vi "ESC controller continuous.vi"() -> ()   [LabVIEW 2020]
panel:
  in  "Max. output (%)":sgl=100.0
  in  "Cool-down time (s)":sgl=60.0
  in  "end":bool
  out "Cool time":sgl(slide) caption="Cooling down...." scale=0.0..1.0
  in  "S-stop":bool
  in  "Output %":sgl(slide) min=0 max=20 scale=0.0..100.0
  in  "E-stop":bool
  out "Error out":errorcluster
  in  "Port":refnum<visa-resource-name>
  # "PN 15/02/2017"
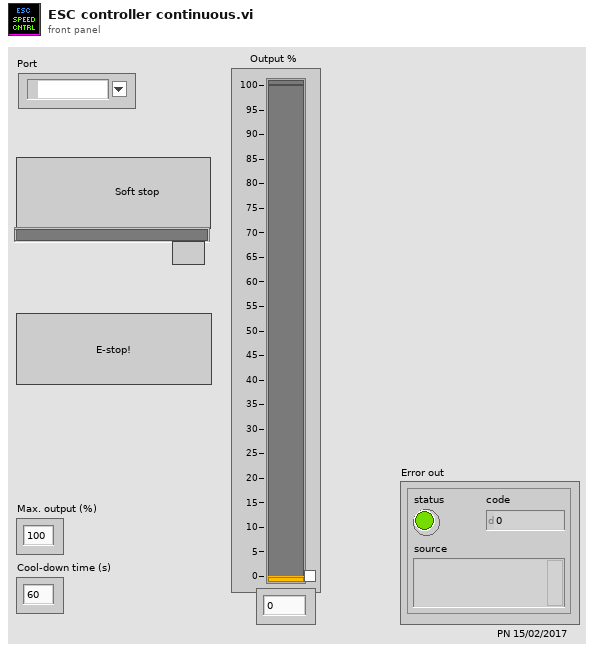
[diagram p1: front panel]
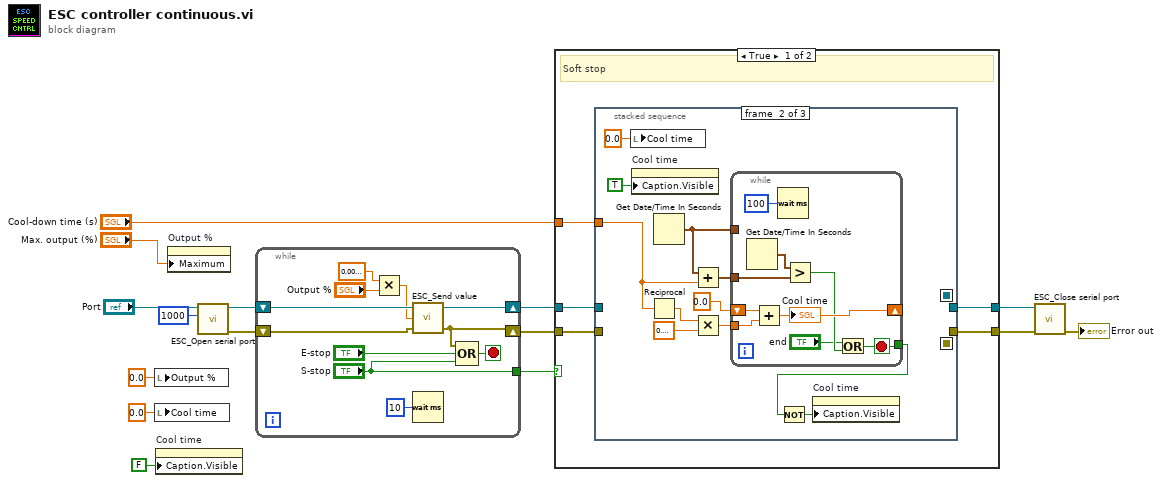
[diagram p0: block diagram]
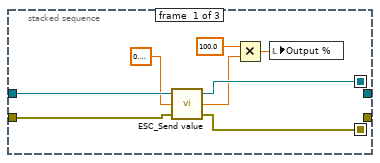
[diagram p2: hidden frame]
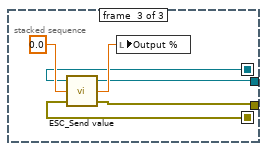
[diagram p3: hidden frame]
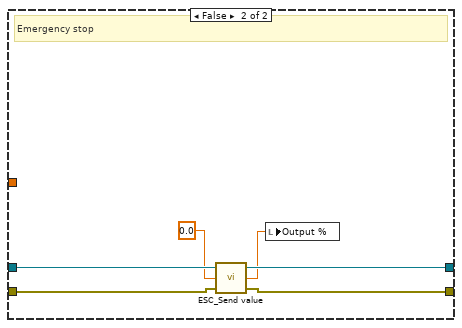
[diagram p4: hidden frame]
diagram:
  n1 = local write "Output %"(sgl 0.0 ("Output %")) -> ()
  n2 = local write "Cool time"(sgl 0.0 ("Cool time")) -> ()
  n3 = property on="Cool time" class="Slide (strict)"("Caption.Visible"=FALSE) -> ()  [unwired: 2 in, 2 out]
  n4 = property on="Output %" class="Slide (strict)"("Maximum"="Max. output (%)") -> ()  [unwired: 2 in, 2 out]
  n5 = call "ESC_Open serial port.vi"("timeout (ms)"=u32 1000, "VISA resource name"="Port") -> ("Error out"=w13:errorcluster, "VISA resource name out"=w12:refnum<visa-resource-name>)  [unwired: 8 in]
  n6 = while {
    shift-right: [w21] -> w11
    shift-left: w13 -> [w26]
    shift-right: [w24] -> w10
    shift-left: w12 -> [w25]
    tunnel: ["S-stop"] -> w5
    stop <- w20 stop-if-true
    n7 = Multiply(x=sgl 0.01, y="Output %") -> (x*y=w16:sgl)
    n8 = call "ESC_Send value.vi"("Error In"=w26, "Output (0...1)"=w16, "Port"=w25) -> ("Error Out"=w21:errorcluster, "Port out"=w24:refnum<visa-resource-name>)  [unwired: 1 out]
    n9 = Wait (ms)(milliseconds to wait=u32 10) -> ()  [unwired: 1 out]
    n10 = Compound Arithmetic op=OR(w21, "E-stop", "S-stop") -> (w20:bool)
  }
  n11 = case shown="True" w5 {
    tunnel: w11 -> [w31 w71]
    tunnel: w10 -> [w30 w70]
    tunnel: [w28 w69] -> w9
    tunnel: [w29 w68] -> w8
    tunnel: "Cool-down time (s)" -> [w27 _]
    frame True {
      # "Soft stop"
      n12 = stacked-sequence {
        seq-local: [w36 _ _] -> [_ _ w62]
        seq-local: [w35 _ _] -> [_ _ w63]
        tunnel: w31 -> [w39 _ _]
        tunnel: w30 -> [w38 _ _]
        tunnel: [_ _ w61] -> w29
        tunnel: [_ _ w60] -> w28
        tunnel: w27 -> [_ w43 _]
        frame #0 {
          n13 = call "ESC_Send value.vi"("Error In"=w39, "Output (0...1)"=sgl 0.1 ("x"), "Port"=w38) -> ("Error Out"=w36:errorcluster, "Output"=w32:sgl, "Port out"=w35:refnum<visa-resource-name>)
          n14 = Multiply(x=sgl 100.0, y=w32) -> (x*y=w33:sgl)
          n15 = local write "Output %"(w33) -> ()
        }
        frame #1 {
          n16 = local write "Cool time"(sgl 0.0 ("Cool time")) -> ()
          n17 = property on="Cool time" class="Slide (strict)"("Caption.Visible"=TRUE) -> ()  [unwired: 2 in, 2 out]
          n18 = Reciprocal(x=w43) -> (1/x=w48:sgl)
          n19 = Get Date/Time In Seconds() -> (seconds since 1Jan1904=w49:timestamp)
          n20 = Add(x=w49, y=w43) -> (x+y=w50:timestamp)
          n21 = Multiply(x=w48, y=sgl 0.1) -> (x*y=w46:sgl)
          n22 = while {
            tunnel: w50 -> [w59]
            tunnel: w49 -> [_]
            tunnel: w46 -> [w55]
            shift-right: [w54] -> _
            shift-left: sgl 0.0 ("y") -> [w56]
            tunnel: [w51] -> w40
            stop <- w51 stop-if-true
            n23 = Get Date/Time In Seconds() -> (seconds since 1Jan1904=w58:timestamp)
            n24 = Add(x=w56, y=w55) -> (x+y=w54:sgl)
            "Cool time" <- w54
            n25 = Wait (ms)(milliseconds to wait=u32 100) -> ()  [unwired: 1 out]
            n26 = Greater?(x=w58, y=w59) -> (0:w53:bool)
            n27 = Or(x="end", y=w53) -> (x .or. y?=w51:bool)
          }
          n28 = Not(x=w40) -> (.not. x?=w41:bool)
          n29 = property on="Cool time" class="Slide (strict)"("Caption.Visible"=w41) -> ()  [unwired: 2 in, 2 out]
        }
        frame #2 {
          n30 = call "ESC_Send value.vi"("Error In"=w62, "Output (0...1)"=sgl 0.0 ("x"), "Port"=w63) -> ("Error Out"=w60:errorcluster, "Output"=w64:sgl, "Port out"=w61:refnum<visa-resource-name>)
          n31 = local write "Output %"(w64) -> ()
        }
      }
    }
    frame False {
      # "Emergency stop"
      n32 = call "ESC_Send value.vi"("Error In"=w71, "Output (0...1)"=sgl 0.0 ("x"), "Port"=w70) -> ("Error Out"=w69:errorcluster, "Output"=w66:sgl, "Port out"=w68:refnum<visa-resource-name>)
      n33 = local write "Output %"(w66) -> ()
    }
  }
  n34 = call "ESC_Close serial port.vi"("Error in"=w9, "VISA resource name"=w8) -> ("Error out"=→"Error out":errorcluster)  [unwired: 9 in]
